vi "Default Settings.vi"(8 "error in (no error)":errorcluster, 11 "Offset Dispense in":refnum<class "Offset Dispense.lvclass">) -> (0 "error out":errorcluster, 3 "Offset Dispense out":refnum<class "Offset Dispense.lvclass">)   [LabVIEW 2019, in "Offset Dispense.lvclass"]
uses:
  Offset Dispense.lvclass
  C:/Users/HEP/Documents/Aerotech gantry/UCSB-Gantry-master-main/V5/Classes/Routine/Dispense/CAD Dispense/CAD Dispense.lvclass
  C:/Users/HEP/Documents/Aerotech gantry/UCSB-Gantry-master-main/V5/Classes/Routine/Dispense/Dispense.lvclass
  CAD Dispense.lvclass/CAD Dispense.ctl
  Read Glue Speed.vi
  Read Move Speed.vi
  CAD Dispense.lvclass
  Dispense.lvclass
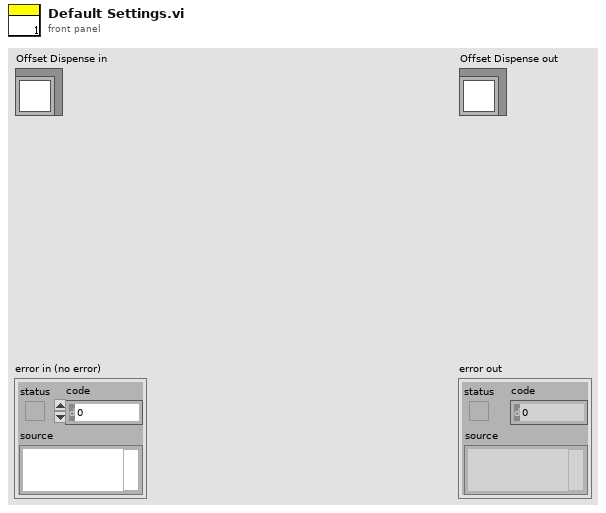
[diagram p1: front panel]
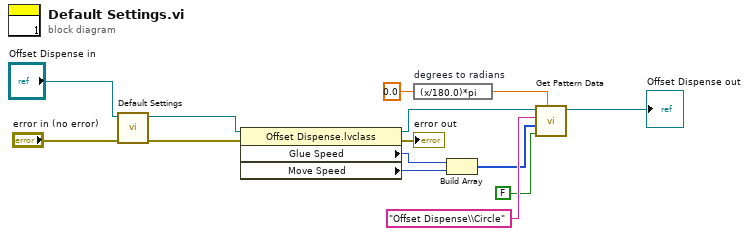
[diagram p0: block diagram]
diagram:
  n1 = call-parent "Default Settings.vi"("error in (no error)"="error in (no error)", "CAD Dispense in"="Offset Dispense in") -> ("error out"=w3:errorcluster, "CAD Dispense out"=w1:refnum<class "Offset Dispense.lvclass">)  [unwired: 8 in]
  n2 = property class="Offset Dispense.lvclass"(reference=w1, error in=w3) -> (reference out=w14:refnum<class "Offset Dispense.lvclass">, error out=→"error out":errorcluster, "Glue Speed"=w7:i32, "Move Speed"=w6:i32)
  n3 = expression code="(x/180.0)*pi" "degrees to radians"(0.0) -> (w11:dbl)
  n4 = Build Array(w7, w6) -> (w8:i32[])
  n5 = call "Get Pattern Data.vi"("theta"=w11, "Iterative?"=FALSE, "File Name"=w8, "Folder Name"="Offset Dispense\\Circle", "Dispense.lvclass"=w14) -> ("Dispense Out"=→"Offset Dispense out":refnum<class "Offset Dispense.lvclass">)  [unwired: 6 in]
